vi "AVI-Load playback parameters.vi"(8 "error in (no error)":errorcluster, 9 "AVI File Path":path=path "D:/Microscope data/10 Sep 2014/TimeLapse 10_09_2014 18-46-40 512x512/Experiment Header.ini", 11 "I16 image ref":T1) -> (0 "error out":errorcluster)   [LabVIEW 2017]
uses:
  <vilib>/vision/Image Controls.llb/IMAQ Image.ctl
  Functional Imaging Viewer/SubVIs/Experiment header interface/Typedefs/Header file interface module functions enum.ctl
  Globals/gl_Time series viewer globals.vi
  Global Variables/General Globals.vi
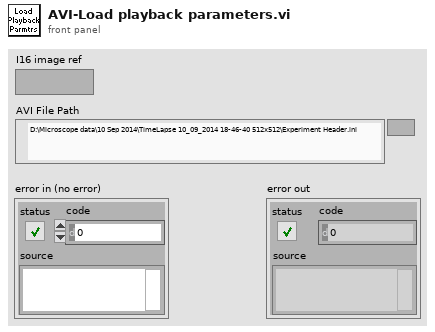
[diagram p1: front panel]
types:
  T1 = typedef "IMAQ Image.ctl" = refnum<image>
  T2 = typedef "Header file interface module functions enum.ctl" = enum16{"Load experiment header file", "Save experiment header file", "Clear stored values", "Read stored values", "Update specific value in memory", "Update values in memory"}
  T3 = typedef "Header parameters cluster-ALL.ctl" = cluster{"LOGIN":T4, "GLOBAL PARAMETERS":T5, "IMAGING MODES":T7, "TIME SERIES":T8, "MOTOR Z-STACK ":T10, "AOL Z-STACK":T11, "FUNCTIONAL IMAGING":T12, "MOVEMENT CORRECTION":T13, "CALIBRATION":T15, "STATISTICS":T16, "BIOLOGY INFORMATION":T17}
  T4 = typedef "Header params -Login.ctl" = cluster{"User":string, "Profile":string, "Software Version":string, "Experiment Date Time":timestamp}
  T5 = typedef "Header params-Global Parameters.ctl" = cluster{"MicroscopeID":string, "Microscope Type":string, "Objective":string, "Field of View (um)":dbl, "Fill time (us)":dbl, "Experiment Type":T6, "Stimuli Trigger":bool, "Speed Logging":bool}
  T6 = typedef "Experiment Type.ctl" = enum16{"In vivo", "In vitro", "Testing", "Calibration", "Other"}
  T7 = typedef "Header params-Imaging Modes.ctl" = cluster{"Time Series":bool, "Motor Zstack":bool, "AOL Zstack":bool, "Functional Imaging":bool}
  T8 = typedef "Header params-Time Series.ctl" = cluster{"Basic Image meta data":T9, "AOL z":dbl}
  T9 = typedef "Header params-Basic image meta data.ctl" = cluster{"Wavelength (nm)":dbl, "# averaged frames":dbl, "laser power (%)":dbl, "Pockels":dbl, "pixel dwell time (us)":dbl, "pmt 1":dbl, "pmt 2":dbl, "back apperture":dbl, "zoom":dbl, "field of view":dbl, "frame size":u16, "AOL x centre":dbl, "AOL y centre":dbl, "Stage x position":dbl, "Stage y position":dbl, "Stage z position":dbl}
  T10 = typedef "Header params-Motor Z-stack.ctl" = cluster{"Hdr Basic Image meta data":T9, "Z Start":dbl, "Z Stop":dbl, "No of Planes":dbl}
  T11 = typedef "Header params-AOL Z-stack.ctl" = cluster{"Hdr Basic Image meta data":T9, "Z Start":dbl, "Z Stop":dbl, "No of Planes":dbl}
  T12 = typedef "Header params-Functional Imaging.ctl" = cluster{"Functional Mode":enum16{"Point", "Line", "Patch", "Plane", "Volume"}, "Pockels Modulation":bool, "Number of pois":dbl, "Number of miniscans":dbl, "Number of cycles":dbl, "Number of trials":dbl, "Miniscan dwell time per pixel (us)":dbl, "Number of pixels in miniscan":dbl, "poi dwell time":dbl, "Rectangle ROI length":dbl, "Rectangle ROI height":dbl, "AOL mode":dbl, "Plane mode":dbl, "video length (sec)":dbl, "Frame rate (fps)":dbl, "Stimuli Timing (usec)":dbl, "Acquisition Length":dbl, "Basic Image meta data":T9, "Z Start (um)":dbl, "Z Stop (um)":dbl}
  T13 = typedef "Header params-Movement correction.ctl" = cluster{"Movement Correction":bool, "Axial Reference":bool, "Reference Size":dbl, "Reference Source":T14, "Reference dwell time (us)":dbl, "Number of Z lines":dbl, "Size of Z pixels":dbl, "Axial Pixels":dbl, "Reference Zoom":dbl, "Reference Average":dbl, "Proportional Scale":dbl, "Integral Scale":dbl, "Proportional Scale Z":dbl, "Integral Scale Z":dbl, "Scan Interval":dbl, "Ref Plot Refresh Rate":dbl}
  T14 = typedef "Reference source.ctl" = enum16{"Green channel", "Red channel"}
  T15 = typedef "Header params-Calibration Setup.ctl" = cluster{"Pockels Calibration File":path, "Calibration_ini file":path, "Setup_ini file":path}
  T16 = typedef "Header params-statistics.ctl" = cluster{"Z-stack duration (sec)":dbl, "Number of acquired data-points":dbl, "Acquisition time (ms)":dbl, "Number of acquired frames":dbl}
  T17 = typedef "Biology Information.ctl" = cluster{"Animal Code or Name":string, "Animal DoB":string, "Animal Age":string, "Animal Sex":string, "Animal Weight":string, "Date of Injection":string, "Date of Implant":string, "Site of Injection":string, "Animal Ear Notch":string, "AAV constructs":string, "Genetic background":string, "Optical reporter":string, "Region of brain imaged":string, "Other \ncomments":string}
  T18 = typedef "AVI playback header info cluster.ctl" = cluster{"Frame Size":u32, "AOD fill time (us)":dbl, "Dwell time (us)":dbl, "Frame period (ms)":dbl, "Number of Miniscans":u16, "Number of Pixels in Miniscan":u16}
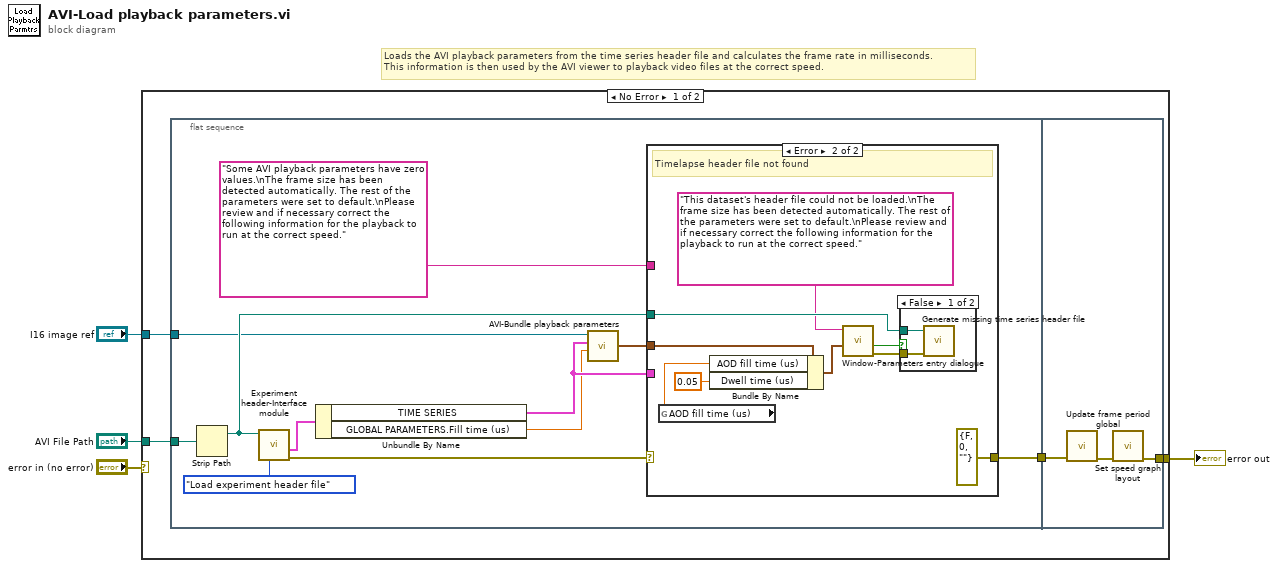
[diagram p0: block diagram]
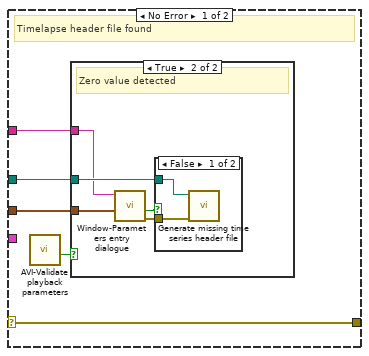
[diagram p2: hidden frame]
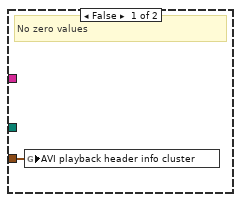
[diagram p3: hidden frame]
diagram:
  # "Loads the AVI playback parameters from the time series header file and calculates the frame rate in milliseconds.\nThis information is then used by the AVI viewer to playback video files at the correct speed."
  n1 = case shown="No Error" "error in (no error)" {
    selector: "error in (no error)" -> [_ w47]
    tunnel: [w6 w47] -> w4
    tunnel: "AVI File Path" -> [w8 _]
    tunnel: "I16 image ref" -> [w5 _]
    frame No Error {
      n2 = flat-sequence {
        tunnel: w8 -> [w19]
        tunnel: [w12] -> w7
        tunnel: w5 -> [w14]
        tunnel: [w44] -> w6
        tunnel: w7 -> [w46]
        frame #0 {
          n3 = Strip Path(path=w19) -> (stripped path=w16:path)  [unwired: 1 out]
          n4 = call "Experiment header-Interface module.vi"("Function"=Header_file_interface_module_functions_enum."Load experiment header file", "Experiment data folder path"=w16) -> ("error out"=w17:errorcluster, "All header parameters out"=w11:T3)  [unwired: 8 in]
          n5 = Unbundle By Name(w11) -> ("TIME SERIES"=w10:T8, "GLOBAL PARAMETERS.Fill time (us)"=w9:dbl)
          n6 = call "AVI-Bundle playback parameters.vi"("Fill time"=w9, "TIME SERIES"=w10, "I16 image ref"=w14) -> ("AVI playback header info cluster"=w15:T18)  [unwired: 8 in]
          n7 = case shown="Error" w17 {
            selector: w17 -> [w20 _]
            tunnel: w10 -> [_ _]
            tunnel: w16 -> [w22 w40]
            tunnel: w15 -> [w23 w36]
            tunnel: "Some AVI playback parameters have zero values.\nThe frame size has been detected automatically. The rest of the parameters were set to default.\nPlease review and if necessary correct the following information for the playback to run at the correct speed." ("Message") -> [w21 _]
            tunnel: [w20 errorcluster {"status"=FALSE, "code"=0, "source"=""} ("error IO")] -> w12
            frame No Error {
              # "Timelapse header file found"
              n8 = call "AVI-Validate playback parameters.vi"() -> ("Zero value detected"=w24:bool)  [unwired: 10 in, 1 out]
              n9 = case shown="True" w24 {
                tunnel: w23 -> [w25 w29]
                tunnel: w22 -> [_ w28]
                tunnel: w21 -> [_ w26]
                frame False {
                  # "No zero values"
                  n10 = global write "gl_Time series viewer globals.vi" "AVI playback header info cluster"(w25) -> ()
                }
                frame True {
                  # "Zero value detected"
                  n11 = call "Window-Parameters entry dialogue.vi"("AVI playback header info cluster"=w29, "Message"=w26) -> ("error out"=w30:errorcluster, "Cancelled"=w27:bool)  [unwired: 8 in]
                  n12 = case shown="False" w27 {
                    tunnel: w30 -> [w32 _]
                    tunnel: w28 -> [w31 _]
                    frame False {
                      n13 = call "Generate missing time series header file.vi"("error in (no error)"=w32, "Timelapse data folder path"=w31) -> ()  [unwired: 10 in]
                    }
                    frame True {
                    }
                  }
                }
              }
            }
            frame Error {
              # "Timelapse header file not found"
              n14 = global read "General Globals.vi" "AOD fill time (us)"() -> (w34:dbl)
              n15 = Bundle By Name(cluster=w36, "AOD fill time (us)"=w34, "Dwell time (us)"=0.05) -> (w37:T18)
              n16 = call "Window-Parameters entry dialogue.vi"("AVI playback header info cluster"=w37, "Message"="This dataset's header file could not be loaded.\nThe frame size has been detected automatically. The rest of the parameters were set to default.\nPlease review and if necessary correct the following information for the playback to run at the correct speed.") -> ("error out"=w41:errorcluster, "Cancelled"=w38:bool)  [unwired: 8 in]
              n17 = case shown="False" w38 {
                tunnel: w41 -> [w43 _]
                tunnel: w40 -> [w42 _]
                frame False {
                  n18 = call "Generate missing time series header file.vi"("error in (no error)"=w43, "Timelapse data folder path"=w42) -> ()  [unwired: 10 in]
                }
                frame True {
                }
              }
            }
          }
        }
        frame #1 {
          n19 = call "Update frame period global.vi"("error in (no error)"=w46) -> ("error out"=w45:errorcluster)  [unwired: 10 in]
          n20 = call "Set speed graph layout.vi"("error in (no error)"=w45) -> ("error out"=w44:errorcluster)  [unwired: 10 in]
        }
      }
    }
    frame Error {
    }
  }
  "error out" <- w4
